vi "Write Labels.vi"(8 "error in (no error)":errorcluster, 10 "Labels":string[](array[string]), 11 "Control Info in":refnum<class "Control Info.lvclass">) -> (0 "error out":errorcluster, 3 "Control Info out":refnum<class "Control Info.lvclass">)   [LabVIEW 2017, in "Localization.lvlib" / "Control Info.lvclass"]
doc: "If the Labels input is empty, writes the Labels that are defined in the Labels [Additional Labels] data from the class data. Otherwise the data in the Labels input is written to the file and the Labels [Additional labels] data in the class data. The data is written to the INI file that is currently in the class data.\n\nChoose Movement Consulting, LLC"
uses:
  Control Info.lvclass
  Control Info.lvclass/Control Info.ctl
  <vilib>/Utility/config.llb/Write Key (String).vi
  <vilib>/Utility/config.llb/NI_LVConfig.lvlib
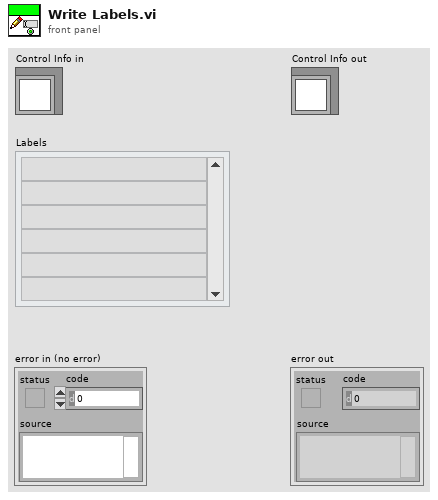
[diagram p1: front panel]
types:
  T1 = typedef "NI_LVConfig.lvlib/Config Data RefNum.ctl" = refnum<k1>
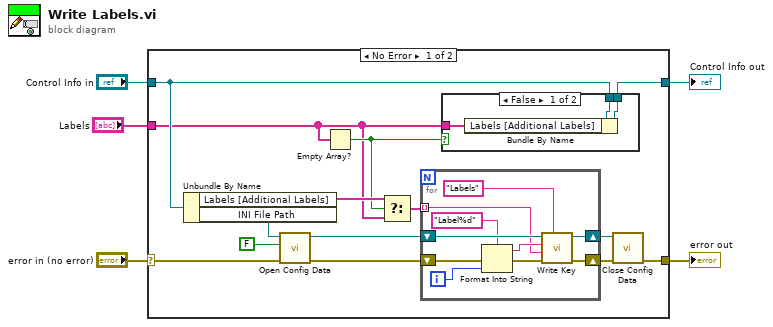
[diagram p0: block diagram]
diagram:
  n1 = case shown="No Error" "error in (no error)" {
    selector: "error in (no error)" -> [w19 w35]
    tunnel: [w14 w35] -> w4
    tunnel: [w9 w34] -> w2
    tunnel: "Control Info in" -> [w8 w34]
    tunnel: "Labels" -> [w6 _]
    frame No Error {
      n2 = Unbundle By Name(w8) -> ("Labels [Additional Labels]"=w11:string[], "INI File Path"=w12:path)
      n3 = call <vilib>:"Open Config Data.vi"("error in (no error)"=w19, "create file if necessary (T)"=FALSE, "configuration file path"=w12) -> ("error out"=w16:errorcluster, "refnum"=w17:T1)  [unwired: 6 in, 1 out]
      n4 = Empty Array?(array=w6) -> (empty?=w7:bool)
      n5 = Select(t=w11, s=w7, f=w6) -> (s? t:f=w10:string[])
      n6 = for {
        shift-right: [w31] -> w15
        shift-left: w16 -> [w29]
        shift-right: [w30] -> w13
        shift-left: w17 -> [w33]
        tunnel: w10 -> [w24] mode=indexing
        i -> [w27]
        n7 = Format Into String(format string="Label%d" ("section"), error in=w29, w27) -> (resulting string=w25:string, error out=w28:errorcluster)  [unwired: 1 in]
        n8 = call-poly <vilib>:"Write Key.vi"("section"="Labels", "error in (no error)"=w28, "value"=w24, "key"=w25, "refnum"=w33) -> ("error out"=w31:errorcluster, "refnum out"=w30:T1)  [unwired: 4 in, 1 out]
      }
      n9 = case shown="False" w7 {
        tunnel: w8 -> [w22 w23]
        tunnel: [w21 w23] -> w9
        tunnel: w6 -> [w20 _]
        frame False {
          n10 = Bundle By Name(cluster=w22, "Labels [Additional Labels]"=w20) -> (w21:refnum<class "Control Info.lvclass">)
        }
        frame True {
        }
      }
      n11 = call <vilib>:"Close Config Data.vi"("error in (no error)"=w15, "refnum"=w13) -> ("error out"=w14:errorcluster)  [unwired: 8 in, 1 out]
    }
    frame Error {
    }
  }
  "error out" <- w4
  "Control Info out" <- w2
